vi "shag_start — 1.vi"() -> ()   [LabVIEW 2016]
uses:
  <vilib>/Instr/_visa.llb/VISA Configure Serial Port (Instr).vi
panel:
  in  "?":T1(tab)
  in  "stop":bool
  in  "Минуты":i32 min=-600 max=11400
  in  "Вращение -":bool
  in  "Вращение +":bool
  in  "Вернуться в нулевое положение":bool
  in  "Задать текущее положение нулевым":bool
  out "Текущее положение\n в минутах":i32
  out "положение шд":i32(knob) scale=-10.0..190.0
  in  "Вращение + 2":bool
  in  "Вращение - 2":bool
  out "текущее положенин":string
  in  "Stop SHAG":bool
  in  "Выберете COM порт":refnum<visa-resource-name>="COM1"
  in  "Скорость обмена данными":u32(ring)=19200 items=["9600"=9600, "19200"=19200, "38400"=38400, "57600"=57600]
  in  "Число бит на символ":u16=8 min=5 max=8 step=1
  in  "Контроль чётности":enum16{"None", "Odd", "Even", "Mark", "Space"}(ring)
  in  "Стоповый бит":u16(ring)=10 items=["1.0"=10, "1.5"=15, "2.0"=20]
  in  "Контроль переполнения":u16(ring) items=["None"=0, "XON/XOFF"=1, "RTS/CTS"=2, "DTR/DSR"=4]
  # "1 - адресс 1 двигателя\n2 - адресс 2 двигателя\n$0MV\\01+   - запуск всех двигателей в положительном направлении \n$0MS\\00   - остановка всех двигателей\n$0MJ\\04+\\00\\00\\01   - 1 шаг всех двигателей\n$0SS\\01\\10   - скорость 10 для всех двигателей"
  # "Положение ШД 0:"
  # "Положение ШД 0 в минутах:"
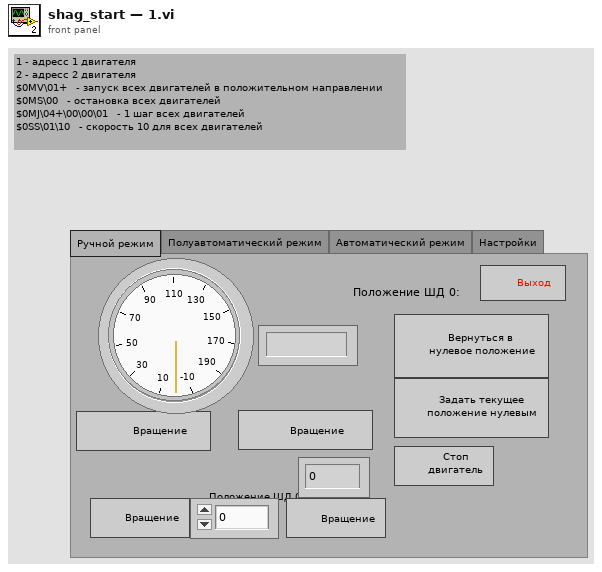
[diagram p1: front panel]
types:
  T1 = enum32{"Ручной режим", "Полуавтоматический режим", "Автоматический режим", "Настройки"}
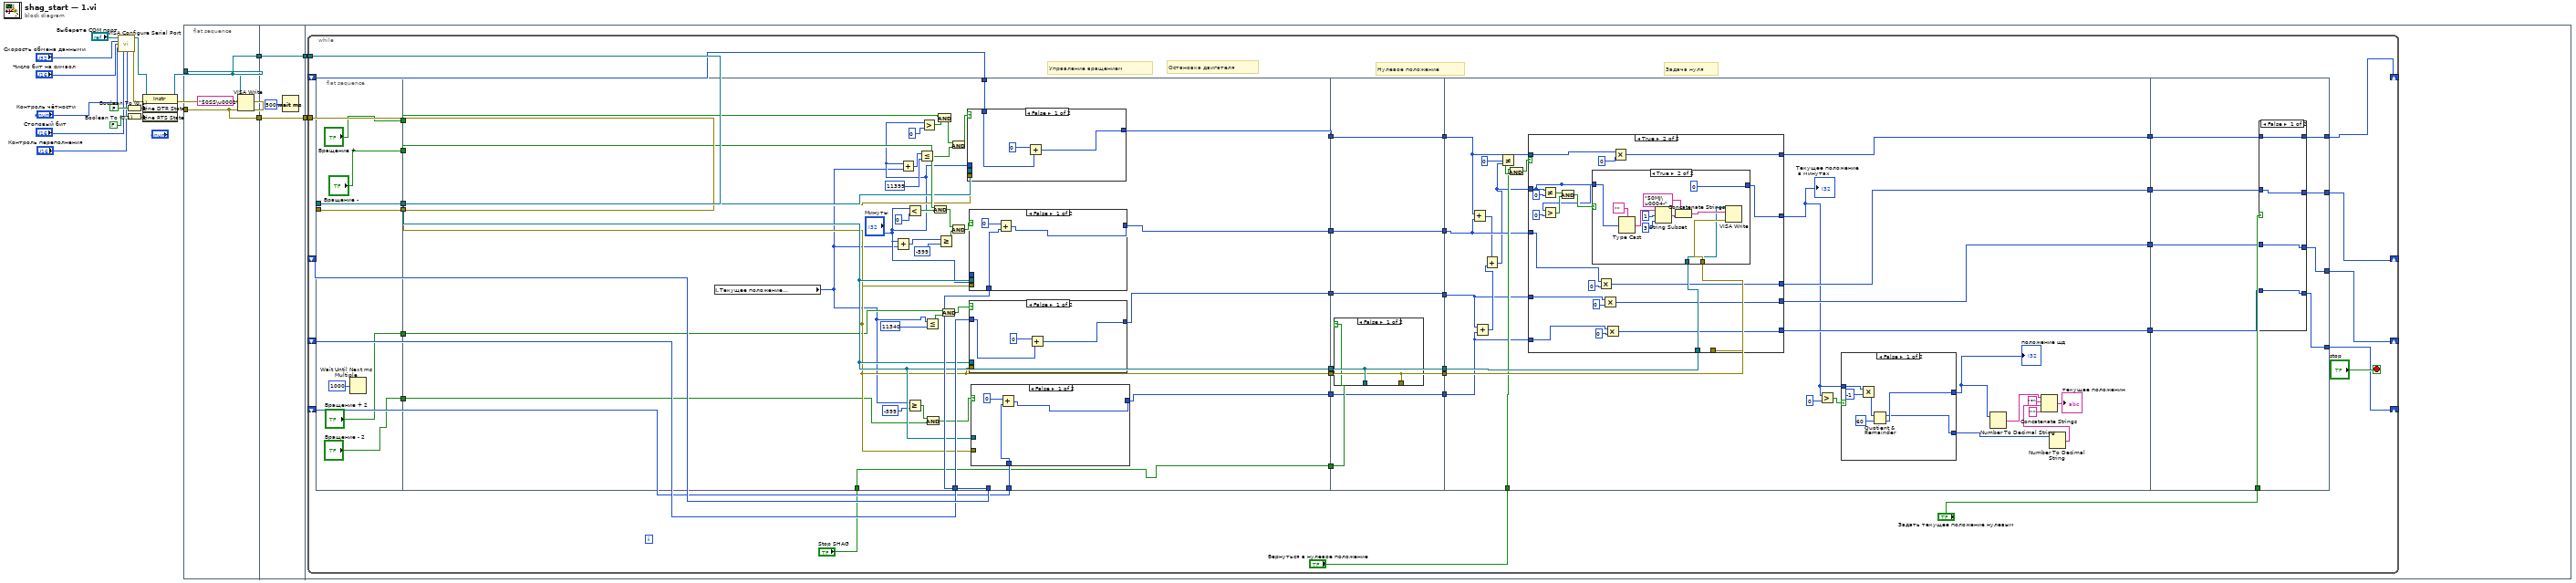
[diagram p0: block diagram]
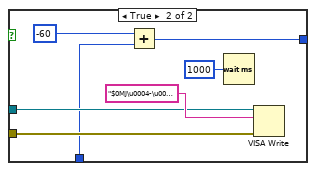
[diagram p2: hidden frame]
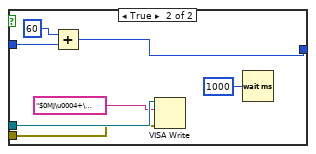
[diagram p3: hidden frame]
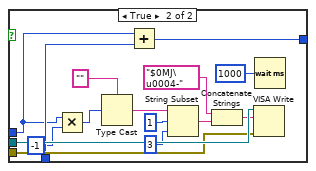
[diagram p4: hidden frame]
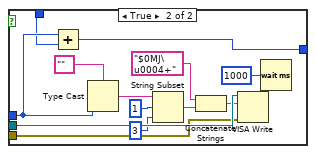
[diagram p5: hidden frame]
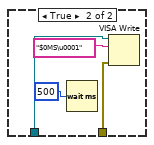
[diagram p6: hidden frame]
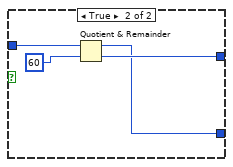
[diagram p7: hidden frame]
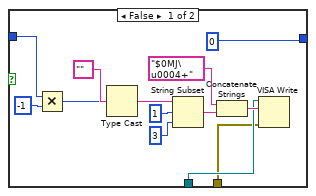
[diagram p9: hidden frame]
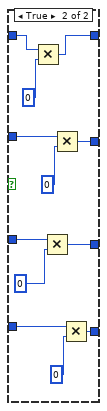
[diagram p10: hidden frame]
diagram:
  n1 = call-poly "VISA Configure Serial Port"("VISA resource name"="Выберете COM порт", "baud rate (9600)"="Скорость обмена данными", "data bits (8)"="Число бит на символ", "parity (0:none)"="Контроль чётности", "stop bits (10: 1 bit)"="Стоповый бит", "flow control (0:none)"="Контроль переполнения") -> ("VISA resource name out"=w16:refnum<visa-resource-name>, "error out"=w15:errorcluster)  [unwired: 8 in]
  n2 = Boolean To (0,1)(Boolean=FALSE ("DTR Write")) -> (0, 1=w17:i16)
  n3 = Boolean To (0,1)(Boolean=FALSE ("DTR Write")) -> (0, 1=w18:i16)
  n4 = property class="Instr"(reference=w16, error in=w15, "Serial Settings:Modem Line Settings:Line DTR State"=w17, "Serial Settings:Modem Line Settings:Line RTS State"=w18) -> (reference out=w14:refnum<visa-resource-name>, error out=w13:errorcluster)
  n5 = flat-sequence {
    tunnel: w14 -> [w20]
    tunnel: w13 -> [w19]
    tunnel: [w20] -> w11
    tunnel: [w19] -> w10
    tunnel: [w23] -> w12
    tunnel: w11 -> [w23]
    tunnel: w10 -> [w22]
    tunnel: [w22] -> w9
    tunnel: w12 -> [w26]
    tunnel: w9 -> [w25]
    frame #0 {
      n6 = VISA Write(VISA resource name=w20, write buffer="$0SS\u0001\u0010", error in (no error)=w19) -> ()  [unwired: 3 out]
    }
    frame #1 {
      n7 = Wait (ms)(milliseconds to wait=u32 500) -> ()  [unwired: 1 out]
    }
    frame #2 {
      n8 = while {
        tunnel: w26 -> [w59]
        tunnel: w25 -> [w58]
        shift-right: [w60] -> _
        shift-left: _ -> [w57]
        shift-right: [w55] -> _
        shift-left: _ -> [w56]
        shift-right: [w35] -> _
        shift-left: _ -> [w40]
        shift-right: [w34] -> _
        shift-left: _ -> [w39]
        stop <- "stop" stop-if-true
        # "Остановка двигателя"
        # "Задача нуля"
        # "Нулевое положение"
        # "Управление вращением"
        n9 = flat-sequence {
          tunnel: w58 -> [w69]
          tunnel: w59 -> [w70]
          tunnel: [w70] -> w62
          tunnel: [w69] -> w61
          tunnel: ["Вращение -"] -> w52
          tunnel: ["Вращение +"] -> w51
          tunnel: ["Вращение + 2"] -> w38
          tunnel: ["Вращение - 2"] -> w37
          tunnel: w62 -> [w96]
          tunnel: w61 -> [w95]
          tunnel: [w107] -> w48
          tunnel: w57 -> [w104]
          tunnel: w56 -> [w106]
          tunnel: [w95] -> w46
          tunnel: [w96] -> w44
          tunnel: [w105] -> w42
          tunnel: w52 -> [w99]
          tunnel: w51 -> [w102]
          tunnel: w40 -> [w97]
          tunnel: w39 -> [w94]
          tunnel: w38 -> [w88]
          tunnel: w37 -> [w86]
          tunnel: [w91] -> w36
          tunnel: [w93] -> w33
          tunnel: [w92] -> w31
          tunnel: "Stop SHAG" -> [w91]
          tunnel: w48 -> [w165]
          tunnel: [w165] -> w47
          tunnel: w46 -> [w167]
          tunnel: [w167] -> w45
          tunnel: w44 -> [w168]
          tunnel: [w168] -> w43
          tunnel: w42 -> [w166]
          tunnel: [w166] -> w41
          tunnel: w36 -> [w164]
          tunnel: w33 -> [w163]
          tunnel: [w163] -> w32
          tunnel: w31 -> [w162]
          tunnel: [w162] -> w30
          tunnel: w47 -> [w191]
          tunnel: w45 -> [w199]
          tunnel: w43 -> [w198]
          tunnel: w41 -> [w190]
          tunnel: [w197] -> w54
          tunnel: [w193] -> w53
          tunnel: "Вернуться в нулевое положение" -> [w192]
          tunnel: w32 -> [w186]
          tunnel: w30 -> [w185]
          tunnel: [w184] -> w29
          tunnel: [w183] -> w28
          tunnel: [w267] -> w60
          tunnel: "Задать текущее положение нулевым" -> [w268]
          tunnel: [w264] -> w55
          tunnel: w54 -> [w266]
          tunnel: w53 -> [w265]
          tunnel: [w263] -> w35
          tunnel: [w262] -> w34
          tunnel: w29 -> [w261]
          tunnel: w28 -> [w260]
          frame #0 {
            n10 = Wait Until Next ms Multiple(millisecond multiple=u32 1000) -> ()  [unwired: 1 out]
          }
          frame #1 {
            n11 = local read "Текущее положение\n в минутах"() -> (w72:i32)
            n12 = Add(x="Минуты", y=w72) -> (x+y=w71:i32)
            n13 = Add(x="Минуты", y=w72) -> (x+y=w75:i32)
            n14 = Less?(x="Минуты", y=0) -> (x < y?=w98:bool)
            n15 = Greater Or Equal?(x=w72, y=-599) -> (x >= y?=w84:bool)
            n16 = Less Or Equal?(x=w75, y=11399) -> (x <= y?=w74:bool)
            n17 = Greater?(x="Минуты", y=0) -> (0:w101:bool)
            n18 = Less Or Equal?(x=w72, y=11340) -> (x <= y?=w83:bool)
            n19 = And(x=w84, y=w86) -> (x .and. y?=w85:bool)
            n20 = And(x=w99, y=w98) -> (x .and. y?=w79:bool)
            n21 = And(x=w102, y=w101) -> (x .and. y?=w81:bool)
            n22 = Greater Or Equal?(x=w71, y=-599) -> (x >= y?=w78:bool)
            n23 = And(x=w88, y=w83) -> (x .and. y?=w87:bool)
            n24 = And(x=w81, y=w74) -> (x .and. y?=w82:bool)
            n25 = And(x=w79, y=w78) -> (x .and. y?=w77:bool)
            n26 = case shown="False" w82 {
              tunnel: w96 -> [_ w161]
              tunnel: w95 -> [_ w160]
              tunnel: "Минуты" -> [_ w152]
              tunnel: [w147 w151] -> w107
              tunnel: w104 -> [w146 w150]
              frame False {
                n27 = Add(x=0, y=w146) -> (x+y=w147:i32)
              }
              frame True {
                n28 = Add(x=w152, y=w150) -> (x+y=w151:i32)
                n29 = Type Cast(type="", x=w152) -> (*(type *) &x=w155:string)
                n30 = String Subset(string=w155, offset (0)=1, length (rest)=3 ("length (rest)")) -> (substring=w154:string)
                n31 = Concatenate Strings("$0MJ\u0004+" ("write buffer"), w154) -> (w158:string)
                n32 = VISA Write(VISA resource name=w161, write buffer=w158, error in (no error)=w160) -> ()  [unwired: 3 out]
                n33 = Wait (ms)(milliseconds to wait=u32 1000) -> ()  [unwired: 1 out]
              }
            }
            n34 = case shown="False" w77 {
              tunnel: w96 -> [_ w145]
              tunnel: w95 -> [_ w144]
              tunnel: "Минуты" -> [_ w133]
              tunnel: [w129 w136] -> w105
              tunnel: w106 -> [w128 w135]
              frame False {
                n35 = Add(x=0, y=w128) -> (x+y=w129:i32)
              }
              frame True {
                n36 = Multiply(x=w133, y=-1) -> (x*y=w134:i32)
                n37 = Type Cast(type="", x=w134) -> (*(type *) &x=w139:string)
                n38 = Add(x=w133, y=w135) -> (x+y=w136:i32)
                n39 = String Subset(string=w139, offset (0)=1, length (rest)=3 ("length (rest)")) -> (substring=w138:string)
                n40 = Concatenate Strings("$0MJ\u0004-" ("write buffer"), w138) -> (w142:string)
                n41 = VISA Write(VISA resource name=w145, write buffer=w142, error in (no error)=w144) -> ()  [unwired: 3 out]
                n42 = Wait (ms)(milliseconds to wait=u32 1000) -> ()  [unwired: 1 out]
              }
            }
            n43 = case shown="False" w87 {
              tunnel: w96 -> [_ w127]
              tunnel: w95 -> [_ w126]
              tunnel: [w119 w125] -> w93
              tunnel: w97 -> [w118 w124]
              frame False {
                n44 = Add(x=0, y=w118) -> (x+y=w119:i32)
              }
              frame True {
                n45 = Add(x=60, y=w124) -> (x+y=w125:i32)
                n46 = VISA Write(VISA resource name=w127, write buffer="$0MJ\u0004+\u0000\u0000<", error in (no error)=w126) -> ()  [unwired: 3 out]
                n47 = Wait (ms)(milliseconds to wait=u32 1000) -> ()  [unwired: 1 out]
              }
            }
            n48 = case shown="False" w85 {
              tunnel: [w109 w117] -> w92
              tunnel: w96 -> [_ w115]
              tunnel: w95 -> [_ w114]
              tunnel: w94 -> [w108 w112]
              frame False {
                n49 = Add(x=0, y=w108) -> (x+y=w109:i32)
              }
              frame True {
                n50 = Add(x=-60, y=w112) -> (x+y=w117:i32)
                n51 = Wait (ms)(milliseconds to wait=u32 1000) -> ()  [unwired: 1 out]
                n52 = VISA Write(VISA resource name=w115, write buffer="$0MJ\u0004-\u0000\u0000<", error in (no error)=w114) -> ()  [unwired: 3 out]
              }
            }
          }
          frame #2 {
            n53 = case shown="False" w164 {
              tunnel: w168 -> [_ w171]
              tunnel: w167 -> [_ w170]
              frame False {
              }
              frame True {
                n54 = Wait (ms)(milliseconds to wait=u32 500) -> ()  [unwired: 1 out]
                n55 = VISA Write(VISA resource name=w171, write buffer="$0MS\u0001", error in (no error)=w170) -> ()  [unwired: 3 out]
              }
            }
          }
          frame #3 {
            n56 = Add(x=w191, y=w190) -> (x+y=w188:i32)
            n57 = Add(x=w186, y=w185) -> (x+y=w189:i32)
            n58 = Add(x=w188, y=w189) -> (x+y=w187:i32)
            n59 = Not Equal?(x=0, y=w187) -> (x != y?=w194:bool)
            n60 = And(x=w192, y=w194) -> (x .and. y?=w196:bool)
            n61 = case shown="True" w196 {
              tunnel: w199 -> [_ w235]
              tunnel: w198 -> [_ w234]
              tunnel: [w214 w233] -> w180
              tunnel: w191 -> [w213 w230]
              tunnel: [w213 w229] -> w197
              tunnel: [w212 w228] -> w193
              tunnel: w190 -> [w212 w224]
              tunnel: w187 -> [w214 w222]
              tunnel: w186 -> [w211 w218]
              tunnel: w185 -> [w210 w217]
              tunnel: [w211 w216] -> w184
              tunnel: [w210 w215] -> w183
              frame False {
              }
              frame True {
                n62 = Not Equal?(x=w222, y=0) -> (x != y?=w226:bool)
                n63 = Greater?(x=w222, y=0) -> (0:w223:bool)
                n64 = And(x=w226, y=w223) -> (x .and. y?=w225:bool)
                n65 = case shown="True" w225 {
                  tunnel: w235 -> [w240 w252]
                  tunnel: w234 -> [w241 w251]
                  tunnel: w222 -> [w238 w250]
                  tunnel: [0 0] -> w233
                  frame False {
                    n66 = Multiply(x=w238, y=-1) -> (x*y=w236:i32)
                    n67 = Type Cast(type="", x=w236) -> (*(type *) &x=w244:string)
                    n68 = String Subset(string=w244, offset (0)=1, length (rest)=3 ("length (rest)")) -> (substring=w243:string)
                    n69 = Concatenate Strings("$0MJ\u0004+" ("write buffer"), w243) -> (w247:string)
                    n70 = VISA Write(VISA resource name=w241, write buffer=w247, error in (no error)=w240) -> ()  [unwired: 3 out]
                  }
                  frame True {
                    n71 = Type Cast(type="", x=w250) -> (*(type *) &x=w255:string)
                    n72 = String Subset(string=w255, offset (0)=1, length (rest)=3 ("length (rest)")) -> (substring=w254:string)
                    n73 = Concatenate Strings("$0MJ\u0004-" ("write buffer"), w254) -> (w258:string)
                    n74 = VISA Write(VISA resource name=w251, write buffer=w258, error in (no error)=w252) -> ()  [unwired: 3 out]
                  }
                }
                n75 = Multiply(x=w224, y=0) -> (x*y=w228:i32)
                n76 = Multiply(x=w218, y=0) -> (x*y=w216:i32)
                n77 = Multiply(x=w217, y=0) -> (x*y=w215:i32)
                n78 = Multiply(x=w230, y=0) -> (x*y=w229:i32)
              }
            }
            "Текущее положение\n в минутах" <- w180
            n79 = Greater?(x=w180, y=0) -> (0:w182:bool)
            n80 = case shown="False" w182 {
              tunnel: w180 -> [w204 w209]
              tunnel: [w205 w207] -> w177
              tunnel: [w200 w206] -> w175
              frame False {
                n81 = Multiply(x=w204, y=-1) -> (x*y=w202:i32)
                n82 = Quotient & Remainder(x=w202, y=60) -> (x-y*floor(x/y)=w200:i32, floor(x/y)=w205:i32)
              }
              frame True {
                n83 = Quotient & Remainder(x=w209, y=60) -> (x-y*floor(x/y)=w206:i32, floor(x/y)=w207:i32)
              }
            }
            "положение шд" <- w177
            n84 = Number To Decimal String(number=w177) -> (decimal integer string=w176:string)  [unwired: 1 in]
            n85 = Number To Decimal String(number=w175) -> (decimal integer string=w174:string)  [unwired: 1 in]
            n86 = Concatenate Strings(w176, "°" ("string"), w174, "'" ("string")) -> (→"текущее положенин":string)
          }
          frame #4 {
            n87 = case shown="False" w268 {
              tunnel: [w272 w283] -> w267
              tunnel: w266 -> [w272 w284]
              tunnel: w265 -> [w271 w280]
              tunnel: [w271 w279] -> w264
              tunnel: [w270 w276] -> w263
              tunnel: [w269 w275] -> w262
              tunnel: w261 -> [w270 w274]
              tunnel: w260 -> [w269 w273]
              frame False {
              }
              frame True {
                n88 = Multiply(x=w284, y=0) -> (x*y=w283:i32)
                n89 = Multiply(x=w274, y=0) -> (x*y=w276:i32)
                n90 = Multiply(x=w280, y=0) -> (x*y=w279:i32)
                n91 = Multiply(x=w273, y=0) -> (x*y=w275:i32)
              }
            }
          }
        }
      }
    }
  }
